vi "Execute.vi"(8 "Error In":errorcluster, 9 "Workspace":T1, 10 "Control In":T2={"I-O.lvclass"=refnum, "Gantry"=refnum, "Dispenser"="COM1"}, 11 "Dispense in":refnum<class "Dispense.lvclass">) -> (0 "Error Out":errorcluster, 2 "Control Out":T2={"I-O.lvclass"=refnum, "Gantry"=refnum, "Dispenser"="COM1"}, 3 "Dispense out":refnum<class "Dispense.lvclass">)   [LabVIEW 2021, in "Dispense.lvclass"]
uses:
  Dispense.lvclass
  Controller/Controllers.ctl
  Controller/I-O/I-O.lvclass
  C:/Program Files (x86)/Aerotech/A3200/LabVIEW/2010/Bin/Aerotech.A3200.dll
  Program Files (x86)/Aerotech/A3200/LabVIEW/2010/Bin/Aerotech.A3200.dll
  Workspace/Workspace.ctl
  Dispense.lvclass/Dispense.ctl
  Controller/Controller.lvclass
  Workspace/Fixture.lvclass
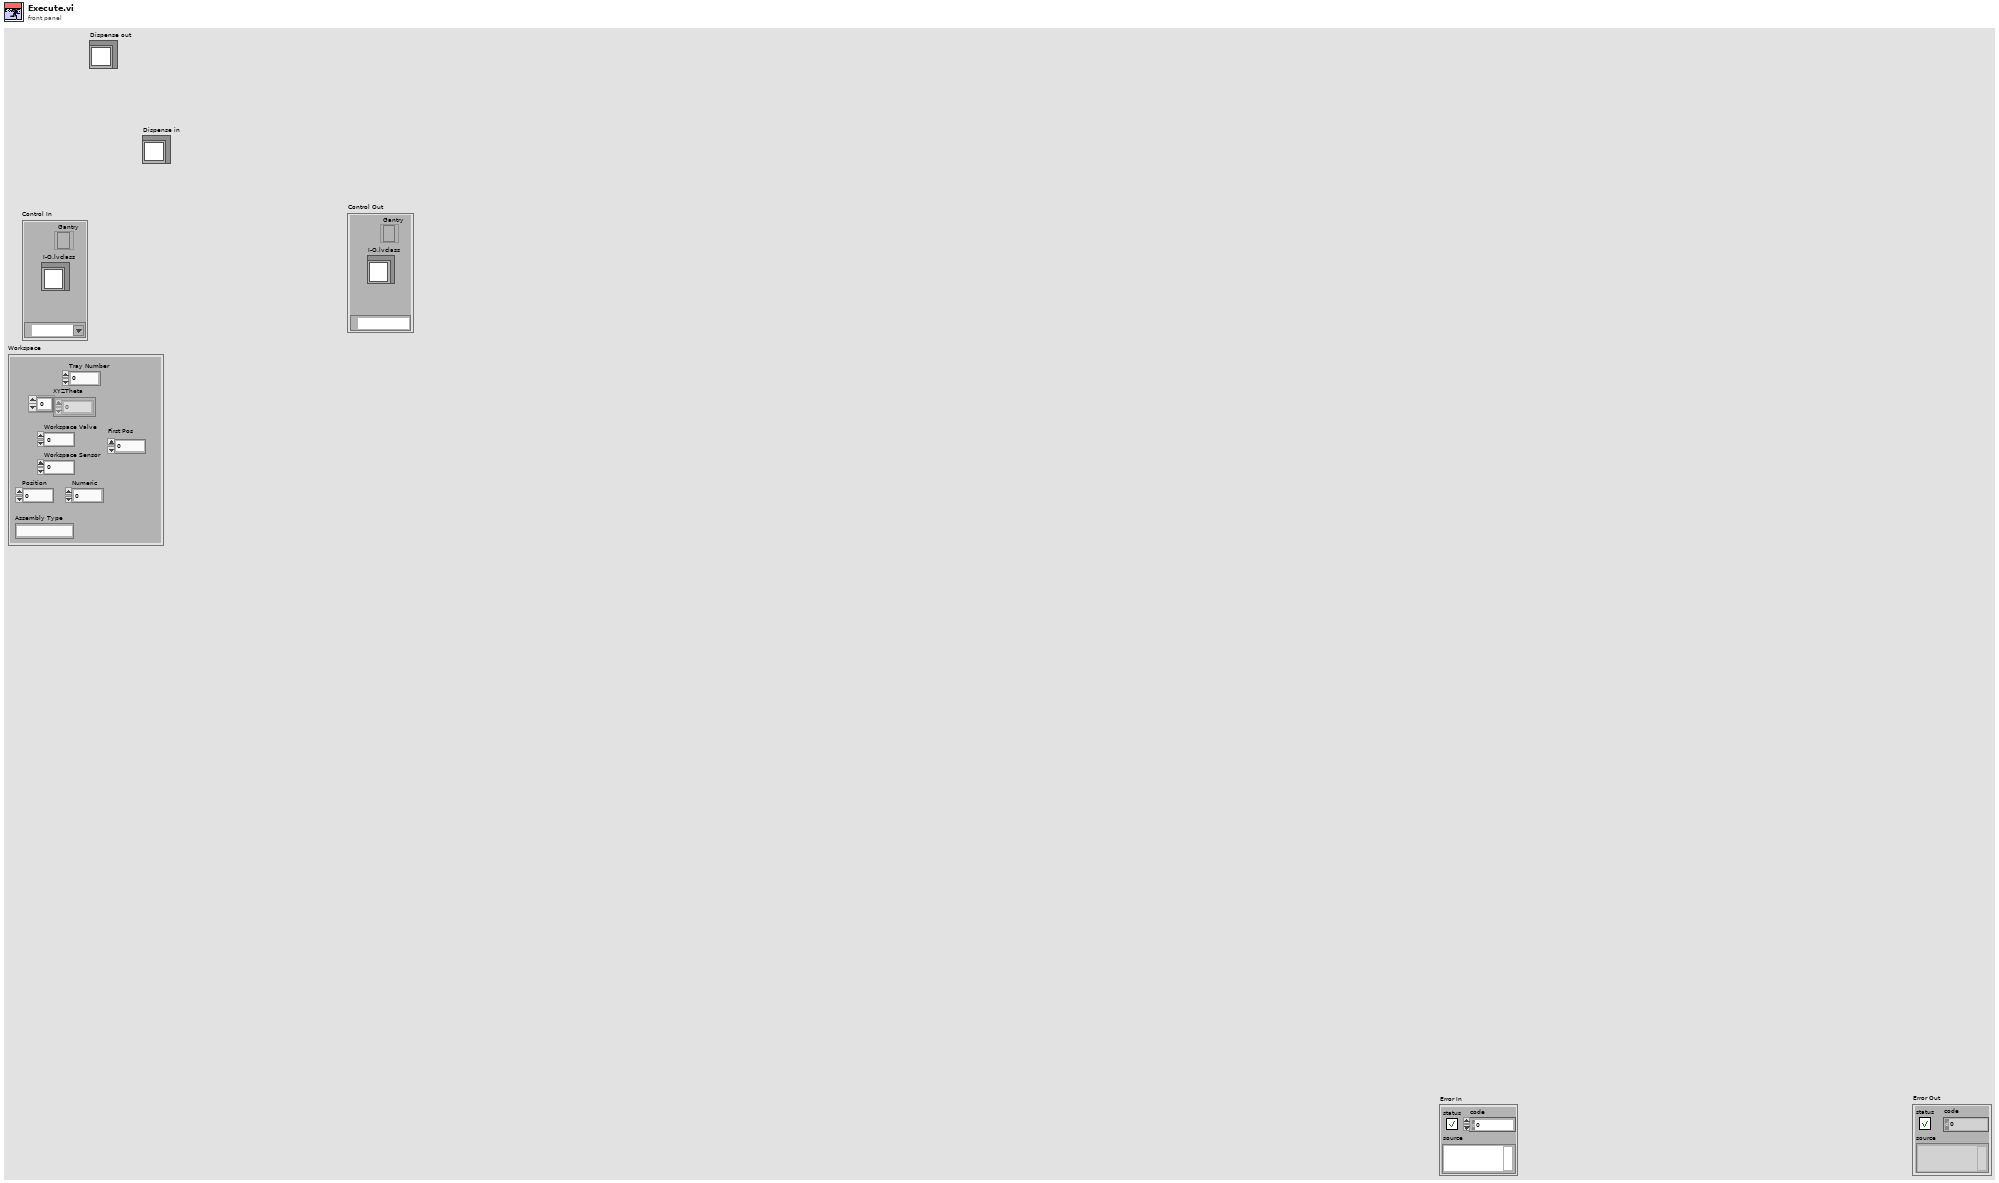
[diagram p1: front panel]
types:
  T1 = typedef "Fixture.lvclass/Workspace.ctl" = cluster{"XYZTheta":dbl[], "Workspace Valve":i32, "Workspace Sensor":i32, "Tray Number":i32, "Position":i32, "Assembly Type":string, "Numeric":dbl, "First Pos":i32}
  T2 = typedef "Controller.lvclass/Controllers.ctl" = cluster{"I-O.lvclass":refnum<class "I-O.lvclass">, "Gantry":refnum<k24>, "Dispenser":refnum<visa-resource-name>}
  T3 = cluster{"Time to Go Down":i32, "Time to Dispense":i32}[]
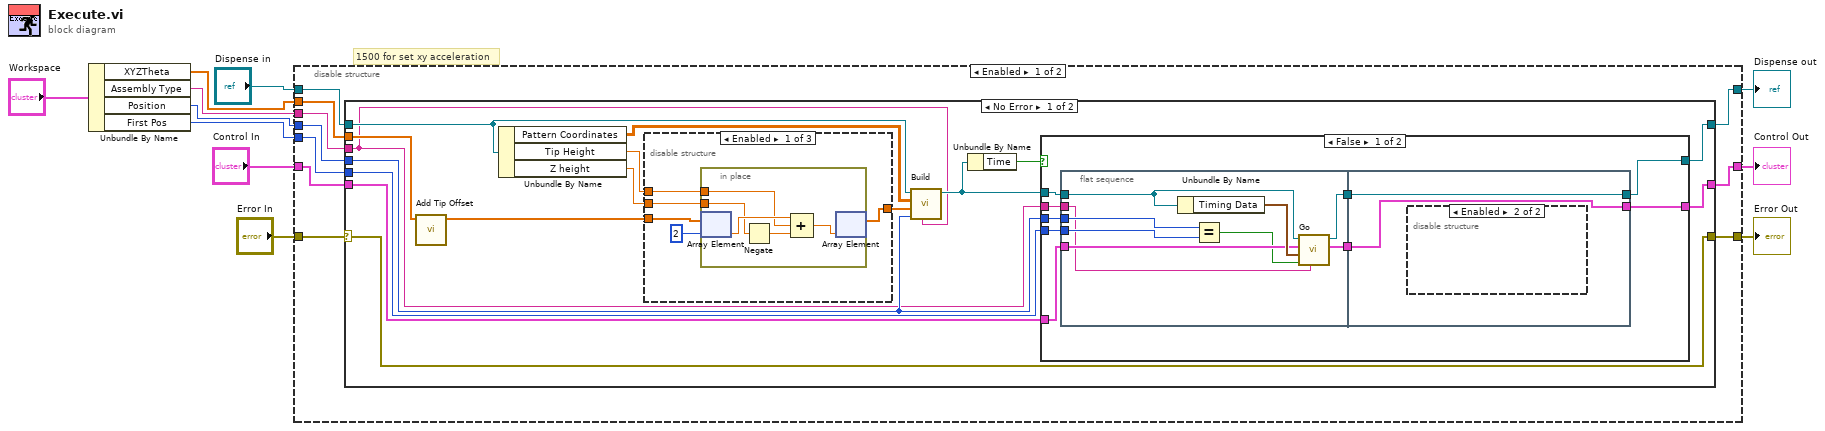
[diagram p0: block diagram]
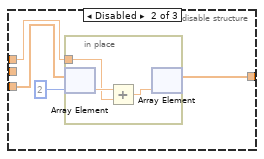
[diagram p2: hidden frame]
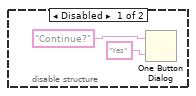
[diagram p4: hidden frame]
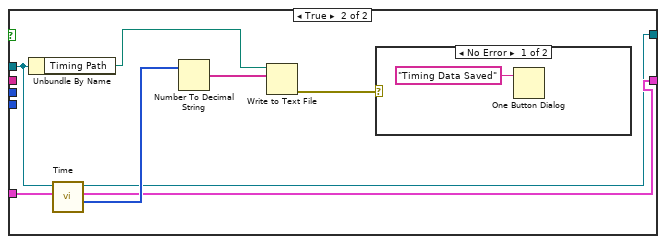
[diagram p5: hidden frame]
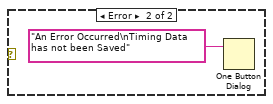
[diagram p6: hidden frame]
diagram:
  # "1500 for set xy acceleration"
  n1 = Unbundle By Name("Workspace") -> ("XYZTheta"=w5:dbl[], "Assembly Type"=w3:string, "Position"=w2:i32, "First Pos"=w1:i32)
  n2 = disable-structure shown="Enabled" {
    disable-tunnel: "Control In" -> [w21 w91]
    disable-tunnel: [w20 w91] -> w10
    disable-tunnel: "Dispense in" -> [w19 w93]
    disable-tunnel: "Error In" -> [w18 w92]
    disable-tunnel: [w17 w92] -> w7
    disable-tunnel: w5 -> [w16 _]
    disable-tunnel: [w15 w93] -> w4
    disable-tunnel: w3 -> [w14 _]
    disable-tunnel: w2 -> [w13 _]
    disable-tunnel: w1 -> [w12 _]
    frame Enabled {
      n3 = case shown="No Error" w18 {
        selector: w18 -> [w37 w89]
        tunnel: w21 -> [w28 w90]
        tunnel: [w27 w90] -> w20
        tunnel: w19 -> [w31 w88]
        tunnel: [w37 w89] -> w17
        tunnel: w16 -> [w26 _]
        tunnel: [w35 w88] -> w15
        tunnel: w14 -> [w23 _]
        tunnel: w13 -> [w24 _]
        tunnel: w12 -> [w25 _]
        frame No Error {
          n4 = call "Add Tip Offset.vi"("XYZTheta"=w26) -> ("XYZTheta"=w30:dbl[])  [unwired: 10 in]
          n5 = Unbundle By Name(w31) -> ("Pattern Coordinates"=w34:dbl[][], "Tip Height"=w32:dbl, "Z height"=w22:dbl)
          n6 = disable-structure shown="Enabled" {
            disable-tunnel: [w41 w50 w55] -> w33
            disable-tunnel: w32 -> [w40 w49 _]
            disable-tunnel: w30 -> [w39 w48 w55]
            disable-tunnel: w22 -> [w38 _ _]
            frame Enabled {
              n7 = in-place {
                in-place-border: w40 -> [w45]
                in-place-border: w38 -> [w44]
                n8 = in-place-array #1(w39, 2) -> (w47:dbl)
                n9 = Negate(x=w44) -> (-x=w43:dbl)
                n10 = Compound Arithmetic op=ADD(w47, w45, w43) -> (w46:dbl)
                n11 = in-place-array #1(w46) -> (w41:dbl[])  [unwired: 1 out]
              }
            }
            frame Disabled {
              n12 = in-place {
                in-place-border: w49 -> [w52]
                n13 = in-place-array #2(w48, 2) -> (w54:dbl)
                n14 = Add(x=w54, y=w52) -> (x+y=w53:dbl)
                n15 = in-place-array #2(w53) -> (w50:dbl[])  [unwired: 1 out]
              }
            }
            frame Disabled {
            }
          }
          n16 = call-dynamic "Build.vi"("Assembly Type"=w23, "Position"=w24, "XYZTheta"=w33, "Pattern Coordinates"=w34, "Dispense in"=w31) -> ("Dispense out"=w36:refnum<class "Dispense.lvclass">)  [unwired: 6 in]
          n17 = Unbundle By Name(w36) -> ("Time"=w29:bool)
          n18 = case shown="False" w29 {
            tunnel: w36 -> [w64 w79]
            tunnel: w28 -> [w63 w81]
            tunnel: [w61 w80] -> w27
            tunnel: [w62 w78] -> w35
            tunnel: w25 -> [w58 _]
            tunnel: w24 -> [w57 _]
            tunnel: w23 -> [w56 _]
            frame False {
              n19 = flat-sequence {
                tunnel: w64 -> [w73]
                tunnel: w63 -> [w69]
                tunnel: [w71] -> w60
                tunnel: [w70] -> w59
                tunnel: w58 -> [w67]
                tunnel: w57 -> [w66]
                tunnel: w56 -> [w65]
                tunnel: [w74] -> w61
                tunnel: [w75] -> w62
                tunnel: w60 -> [w75]
                tunnel: w59 -> [w74]
                frame #0 {
                  n20 = Unbundle By Name(w73) -> ("Timing Data"=w72:T3)
                  n21 = Equal?(x=w66, y=w67) -> (x = y?=w68:bool)
                  n22 = call-dynamic "Go.vi"("assembly type"=w65, "First?"=w68, "Timing Data"=w72, "Control In"=w69, "Dispense in"=w73) -> ("Control Out"=w70:T2, "Dispense Out"=w71:refnum<class "Dispense.lvclass">)  [unwired: 5 in]
                }
                frame #1 {
                  n23 = disable-structure shown="Enabled" {
                    frame Disabled {
                      n24 = One Button Dialog(message="Continue?", button name ("OK")="Yes") -> ()  [unwired: 1 out]
                    }
                    frame Enabled {
                    }
                  }
                }
              }
            }
            frame True {
              n25 = Unbundle By Name(w79) -> ("Timing Path"=w83:path)
              n26 = call-dynamic "Time.vi"("Control In"=w81, "Dispense in"=w79) -> ("Timing Data"=w82:i32[], "Control Out"=w80:T2, "Dispense out"=w78:refnum<class "Dispense.lvclass">)  [unwired: 6 in, 1 out]
              n27 = Number To Decimal String(number=w82) -> (decimal integer string=w84:string[])  [unwired: 1 in]
              n28 = Write to Text File(file (use dialog)=w83, text=w84) -> (error out=w85:errorcluster)  [unwired: 2 in, 2 out]
              n29 = case shown="No Error" w85 {
                frame No Error {
                  n30 = One Button Dialog(message="Timing Data Saved") -> ()  [unwired: 1 in, 1 out]
                }
                frame Error {
                  n31 = One Button Dialog(message="An Error Occurred\nTiming Data has not been Saved") -> ()  [unwired: 1 in, 1 out]
                }
              }
            }
          }
        }
        frame Error {
        }
      }
    }
    frame Disabled {
    }
  }
  "Control Out" <- w10
  "Error Out" <- w7
  "Dispense out" <- w4
